vi "get current activity.vi"(8 "error in (no error)":errorcluster, 11 "Autofocus in":refnum<class "Autofocus.lvclass">) -> (0 "error out":errorcluster, 2 "Current activity":T1=enum."Idle", 3 "Autofocus out":refnum<class "Autofocus.lvclass">)   [LabVIEW 2012, in "Autofocus.lvclass"]
uses:
  Autofocus.lvclass
  current activity.ctl
  Autofocus.lvclass/Autofocus.ctl
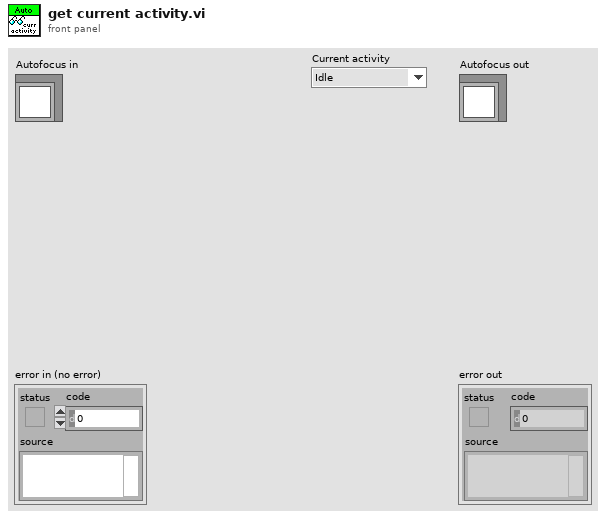
[diagram p1: front panel]
types:
  T1 = typedef "Autofocus.lvclass/current activity.ctl" = enum16{"Image acquisition", "Stack", "Checkpoint", "Idle"}
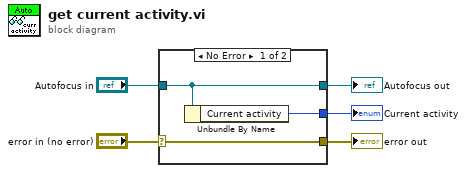
[diagram p0: block diagram]
diagram:
  n1 = case shown="No Error" "error in (no error)" {
    selector: "error in (no error)" -> [w8 w10]
    tunnel: [w8 w10] -> w4
    tunnel: [w7 w9] -> w2
    tunnel: "Autofocus in" -> [w7 w9]
    tunnel: [w6 _] -> w1
    frame No Error {
      n2 = Unbundle By Name(w7) -> ("Current activity"=w6:T1)
    }
    frame Error {
    }
  }
  "error out" <- w4
  "Autofocus out" <- w2
  "Current activity" <- w1
